vi "VI Server_TREE_GetActiveCellString.vi"(4 "Active Cell:Column Number":i32, 6 "Tree.Row.Header":string, 7 "Tree.Label":string, 8 "error in (no error)":errorcluster, 9 "TreeControl in":refnum<vi>, 11 "VI Server.RefsCluster":T1) -> (0 "error out":errorcluster, 1 "TreeControl out":refnum<vi>, 2 "Active Cell:String":string, 3 "VI Server.RefsCluster.DUP":T1={"Labels"=["Tab.Main", "EXIT", "Test.Start", "Test.ABORT", "Test.Pause", "error in", "error out", "Login.Level", "Login.Name", "TestConfiguration.TestCaseEdit", "TestConfiguration.DeleteTestCase", "TestConfiguration.P/N.TestCaseNew", "TestConfiguration.SaveTestCase", "Settings.TestCase.Refresh", "Help", "System.Message", "Instruments.Status", "Test.Tree", "Serial#", "Test.P/N", "Messages & Status", "Settings.P/N", "TestCase", "TestConfiguration", "TestCase.Description", "TestCase.Conditions", "TestCase.Parameter", "TestCaseConfiguration", "TestCase.TraceLimits", "TestCase.Function", "TestCase.Function.Argument1", "TestCase.Function.Argument2", "TestCase.Function.Argument3", "TestCase.Function.Argument3.DBL", "TestCase.LimitsIndex", "LimitsIndex.New", "Limit.Hi", "Limit.Lo", "Limit.Units", "Limits.SAVE", "Limits.Remove", "TestCase.Instrument.Data", "TestCase.InstrumentData.InRange", "TestCase.Execute.Selected", "TestCase.Execute.All", "TestCase.Execute.Pause", "TestCase.Execute.ABORT", "TestCase.Execute.Instruction", "TestCase.Add.Instruction", "TestCase.SAVE", "TestCase.Instrument.Data.Array", "TestCase.Execution.StepTime", "TestCase.Update.Instruction", "Limit.Message", "TestCase.Execute.Pass/Fail", "Performance.Verification.Pass/Fail", "Performance.Verification.SAVE", "TestCase.Execute.Next", "TestConfiguration.RunAll", "TestConfiguration.Execute.Pass/Fail", "TestCaseExecution.StopOnFailure", "TestConfiguration.Run.Step", "TestCase.Add.Instruction.Pos", "TestCase.Execute.Steps", "TestCase.Execute.Step.Pause", "Graph1", "Graph2", "Image1", "Image2", "Image3", "Mem1", "Mem2", "Mem3", "Mem4", "Mem5", "Mem6", "Mem7", "Mem8", "Mem9", "Mem10", "Mem11", "Mem12", "Mem13", "Mem14", "Mem15", "Mem16", "Mem97", "Mem98", "Mem99", "Mem100", "Mem101", "Mem102", "Mem103", "Mem104", "Mem105", "Mem106", "Mem107", "Mem108", "Mem109", "Mem110", "Mem111", "Mem112", "Mem17", "Mem18", "Mem19", "Mem20", "Mem21", "Mem22", "Mem23", "Mem24", "Mem25", "Mem26", "Mem27", "Mem28", "Mem29", "Mem30", "Mem31", "Mem32", "Mem113", "Mem114", "Mem115", "Mem116", "Mem117", "Mem118", "Mem119", "Mem120", "Mem121", "Mem122", "Mem123", "Mem124", "Mem125", "Mem126", "Mem127", "Mem128", "Mem33", "Mem34", "Mem35", "Mem36", "Mem37", "Mem38", "Mem39", "Mem40", "Mem41", "Mem42", "Mem43", "Mem44", "Mem45", "Mem46", "Mem47", "Mem48", "Mem129", "Mem130", "Mem131", "Mem132", "Mem133", "Mem134", "Mem135", "Mem136", "Mem137", "Mem138", "Mem139", "Mem140", "Mem141", "Mem142", "Mem143", "Mem144", "Mem49", "Mem50", "Mem51", "Mem52", "Mem53", "Mem54", "Mem55", "Mem56", "Mem57", "Mem58", "Mem59", "Mem60", "Mem61", "Mem62", "Mem63", "Mem64", "Mem145", "Mem146", "Mem147", "Mem148", "Mem149", "Mem150", "Mem151", "Mem152", "Mem153", "Mem154", "Mem155", "Mem156", "Mem157", "Mem158", "Mem159", "Mem160", "Mem65", "Mem66", "Mem67", "Mem68", "Mem69", "Mem70", "Mem71", "Mem72", "Mem73", "Mem74", "Mem75", "Mem76", "Mem77", "Mem78", "Mem79", "Mem80", "Mem161", "Mem162", "Mem163", "Mem164", "Mem165", "Mem166", "Mem167", "Mem168", "Mem169", "Mem170", "Mem171", "Mem172", "Mem173", "Mem174", "Mem175", "Mem176", "Mem81", "Mem82", "Mem83", "Mem84", "Mem85", "Mem86", "Mem87", "Mem88", "Mem89", "Mem90", "Mem91", "Mem92", "Mem93", "Mem94", "Mem95", "Mem96", "Mem177", "Mem178", "Mem179", "Mem180", "Mem181", "Mem182", "Mem183", "Mem184", "Mem185", "Mem186", "Mem187", "Mem188", "Mem189", "Mem190", "Mem191", "Mem192", "System.SupportedPartNumbers", "System.PartNumber", "System.Instruments", "System.NewInstrument.Name", "System.NewInstrument.Tag", "System.NewInstrument.Path", "UDP.IP.Address", "UDP.LocalPort", "UDP.Port.BC", "UDP.Port.RT", "UDP.Test.String", "UDP.Responce.String", "UDP.Responce.String.Monitor", "UDP.Test.String.Send", "Instr.Responce.Timeout", "UDP.Sent.String", "Performance.Verification.Enable", "UDP.Responce.Array", "UDP.Write.Array", "TestCase.Diagnostics.ABORT", "TestCase.Diagnostics.Pause", "TestCase.Diagnostics.Next", "TestCase.Diagnostics.Instruction", "InstrumentLoad.Disable"], "Refs"=[refnum, refnum, refnum, refnum, refnum, refnum, refnum, refnum, refnum, refnum, refnum, refnum, refnum, refnum, refnum, refnum, refnum, refnum, refnum, refnum, refnum, refnum, refnum, refnum, refnum, refnum, refnum, refnum, refnum, refnum, refnum, refnum, refnum, refnum, refnum, refnum, refnum, refnum, refnum, refnum, refnum, refnum, refnum, refnum, refnum, refnum, refnum, refnum, refnum, refnum, refnum, refnum, refnum, refnum, refnum, refnum, refnum, refnum, refnum, refnum, refnum, refnum, refnum, refnum, refnum, refnum, refnum, refnum, refnum, refnum, refnum, refnum, refnum, refnum, refnum, refnum, refnum, refnum, refnum, refnum, refnum, refnum, refnum, refnum, refnum, refnum, refnum, refnum, refnum, refnum, refnum, refnum, refnum, refnum, refnum, refnum, refnum, refnum, refnum, refnum, refnum, refnum, refnum, refnum, refnum, refnum, refnum, refnum, refnum, refnum, refnum, refnum, refnum, refnum, refnum, refnum, refnum, refnum, refnum, refnum, refnum, refnum, refnum, refnum, refnum, refnum, refnum, refnum, refnum, refnum, refnum, refnum, refnum, refnum, refnum, refnum, refnum, refnum, refnum, refnum, refnum, refnum, refnum, refnum, refnum, refnum, refnum, refnum, refnum, refnum, refnum, refnum, refnum, refnum, refnum, refnum, refnum, refnum, refnum, refnum, refnum, refnum, refnum, refnum, refnum, refnum, refnum, refnum, refnum, refnum, refnum, refnum, refnum, refnum, refnum, refnum, refnum, refnum, refnum, refnum, refnum, refnum, refnum, refnum, refnum, refnum, refnum, refnum, refnum, refnum, refnum, refnum, refnum, refnum, refnum, refnum, refnum, refnum, refnum, refnum, refnum, refnum, refnum, refnum, refnum, refnum, refnum, refnum, refnum, refnum, refnum, refnum, refnum, refnum, refnum, refnum, refnum, refnum, refnum, refnum, refnum, refnum, refnum, refnum, refnum, refnum, refnum, refnum, refnum, refnum, refnum, refnum, refnum, refnum, refnum, refnum, refnum, refnum, refnum, refnum, refnum, refnum, refnum, refnum, refnum, refnum, refnum, refnum, refnum, refnum, refnum, refnum, refnum, refnum, refnum, refnum, refnum, refnum, refnum, refnum, refnum, refnum, refnum, refnum, refnum, refnum, refnum, refnum, refnum, refnum, refnum, refnum, refnum, refnum, refnum, refnum, refnum, refnum, refnum, refnum, refnum, refnum, refnum, refnum, refnum, refnum], "VI Ref"=refnum})   [LabVIEW 2020]
uses:
  VI Server_TypeDefs/VI Server_RefsCluster.ctl
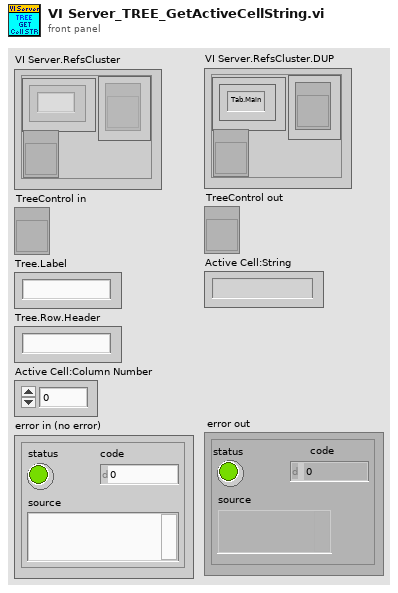
[diagram p1: front panel]
types:
  T1 = typedef "VI Server_RefsCluster.ctl" = cluster{"Labels":string[], "Refs":refnum<vi>[], "VI Ref":refnum<vi>}
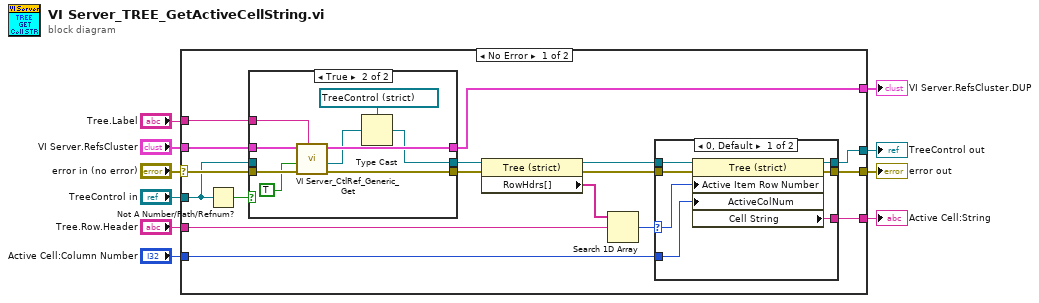
[diagram p0: block diagram]
diagram:
  n1 = case shown="No Error" "error in (no error)" {
    selector: "error in (no error)" -> [w27 w49]
    tunnel: [w15 w49] -> w10
    tunnel: "VI Server.RefsCluster" -> [w26 _]
    tunnel: [w25 _] -> w4
    tunnel: "Tree.Label" -> [w24 _]
    tunnel: [w17 _] -> w3
    tunnel: "Tree.Row.Header" -> [w19 _]
    tunnel: "TreeControl in" -> [w13 _]
    tunnel: "Active Cell:Column Number" -> [w12 _]
    tunnel: [w11 _] -> w7
    frame No Error {
      n2 = Not A Number/Path/Refnum?(number/path/refnum=w13) -> (NaN/Path/Refnum?=w23:bool)
      n3 = case shown="True" w23 {
        tunnel: w27 -> [w39 w48]
        tunnel: w26 -> [w38 w47]
        tunnel: [w38 w46] -> w25
        tunnel: w24 -> [_ w45]
        tunnel: [w39 w43] -> w22
        tunnel: [w37 w42] -> w21
        tunnel: w13 -> [w37 _]
        frame False {
        }
        frame True {
          n4 = call "VI Server_CtlRef_Generic_Get.vi"("Control.Label"=w45, "error in"=w48, "SingleInstance"=TRUE, "VI Server.RefsCluster"=w47) -> ("error out"=w43:errorcluster, "Control.Ref.Generic"=w44:refnum<vi>, "VI Server.RefsCluster.DUP"=w46:T1)  [unwired: 5 in]
          n5 = Type Cast(type=refnum<vi> refnum ("Test.Tree"), x=w44) -> (*(type *) &x=w42:refnum<vi>)
        }
      }
      n6 = property class="Tree (strict)"(reference=w21, error in=w22) -> (reference out=w18:refnum<vi>, error out=w16:errorcluster, "RowHdrs[]"=w20:string[])
      n7 = Search 1D Array(1D array=w20, element=w19) -> (index of element=w14:i32)  [unwired: 1 in]
      n8 = case shown="0, Default" w14 {
        selector: w14 -> [w30 _]
        tunnel: w18 -> [w34 w35]
        tunnel: [w33 w35] -> w17
        tunnel: w16 -> [w32 w36]
        tunnel: [w31 w36] -> w15
        tunnel: w12 -> [w29 _]
        tunnel: [w28 _] -> w11
        frame 0, Default {
          n9 = property class="Tree (strict)"(reference=w34, error in=w32, "Active Item Row Number"=w30, "ActiveColNum"=w29) -> (reference out=w33:refnum<vi>, error out=w31:errorcluster, "Cell String"=w28:string)
        }
        frame -1 {
        }
      }
    }
    frame Error {
    }
  }
  "error out" <- w10
  "TreeControl out" <- w3
  "VI Server.RefsCluster.DUP" <- w4
  "Active Cell:String" <- w7
